vi "Engine - Generic - High Pressure Common Rail Host.vi"() -> ()   [LabVIEW 2015, in "ECS-Host.lvlib"]
uses:
  ECS-Host.lvlib
  <vilib>/addons/Software Calibration Management/XControls/SubHost.xctl
panel:
  out "RailP":sgl caption="[bar]" min=0 max=0.2 step=0.001 format="%#.3f"
  out "RailPStp":sgl caption="[bar]" min=0 max=0.2 step=0.001 format="%#.3f"
  in  "LowsideVoltageSource":enum32{"IMV PID Mode", "12V Puls Power Supply"}(ring)
  in  "_IMV/HPV Tab Control":enum32{"IMV PID", "HPV PID"}(tab)
  in  "IMV_NonPIDFF":sgl caption="[]" format="%#.2f"
  out "IMV_PIDOut":sgl caption="[]" max=50
  in  "IMV_PIDFF":sgl caption="[]" format="%#.2f"
  in  "IMV_Kp":sgl caption="[%/bar]" format="%#.2f"
  in  "IMV_Ti":sgl caption="[]" format="%#.2f"
  in  "IMV_Td":sgl caption="[]" format="%#.2f"
  in  "IMV_PIDMax":sgl caption="[%]" max=50 format="%#.2f"
  in  "IMV_PIDMin":sgl caption="[]" format="%#.2f"
  out "IMV_KpOut":sgl(slide) caption="IMV_ Kc Action" max=0 scale=0.0..100.0 scale format="%#.2f"
  out "IMV_TiOut":sgl(slide) caption="IMV_ Ti Action" max=0 scale=0.0..100.0 scale format="%#.2f"
  out "IMV_TdOut":sgl(slide) caption="IMV_ Td Action" max=0 scale=0.0..100.0 scale format="%#.2f"
  in  "HPV_NonPIDFF":sgl caption="[]" format="%#.2f"
  out "HPV_PIDOut":sgl caption="[]" max=50
  in  "HPV_PIDFF":sgl caption="[]" format="%#.2f"
  in  "HPV_Kp":sgl caption="[%/bar]" format="%#.2f"
  in  "HPV_Ti":sgl caption="[]" format="%#.2f"
  in  "HPV_Td":sgl caption="[]" format="%#.2f"
  in  "HPV_PIDMax":sgl caption="[%]" max=50 format="%#.2f"
  in  "HPV_PIDMin":sgl caption="[]" format="%#.2f"
  out "HPV_KpOut":sgl(slide) caption="HPV_ Kc_Action" max=0 scale=0.0..100.0 scale format="%#.2f"
  out "HPV_TiOut":sgl(slide) caption="IMV_ Ti Action" max=0 scale=0.0..100.0 scale format="%#.2f"
  out "HPV_TdOut":sgl(slide) caption="IMV_ Td Action" max=0 scale=0.0..100.0 scale format="%#.2f"
  in  "RPC Plot":T1(xcontrol)
  in  "IMVDutyCyc_Max":sgl caption="[]" format="%#.2f"
  in  "HPVDutyCyc_Max":sgl caption="[]" format="%#.2f"
  out "BattV":sgl caption="[]" min=0 max=0.2 step=0.001 format="%#.3f"
  out "RailP_Fault":bool
  in  "HPVDutyCyc_Man":sgl caption="[]" format="%#.2f"
  in  "IMVDutyCyc_Man":sgl caption="[]" format="%#.2f"
  in  "IMVDutyCyc_ManE":bool
  out "IMVCurrent_Calc":sgl caption="[]" min=0 max=0.2 step=0.001 format="%#.3f"
  out "IMVDutyCyc_Des":sgl=0.7671859 caption="[]" format="%#.3g"
  in  "IMVDutyCyc_Min":sgl caption="[]" format="%#.2f"
  out "IMVDutyCyc_MaxCalc":sgl caption="[]" max=50 format="%#.3g"
  in  "IMVNomResistance":sgl caption="[]" format="%#.2f"
  in  "IMVPWMFreq":sgl caption="[]" format="%#.2f"
  in  "IMVCtrl_E":bool
  in  "HPVDutyCyc_ManE":bool
  out "HPVCurrent_Calc":sgl caption="[]" min=0 max=0.2 step=0.001 format="%#.3f"
  in  "RailP_MaxThresh":sgl caption="[bar]" min=0 max=0.2 step=0.001 format="%#.3f"
  out "HPVDutyCyc_Des":sgl=0.7671859 caption="[]" format="%#.3g"
  in  "HPVDutyCyc_Min":sgl caption="[]" format="%#.2f"
  out "HPVDutyCyc_MaxCalc":sgl caption="[]" max=50 format="%#.3g"
  in  "HPVNomResistance":sgl caption="[]" format="%#.2f"
  in  "HPVPWMFreq":sgl caption="[Hz]" format="%#.2f"
  in  "HPVCtrl_E":bool
  in  "RailPControlMode":enum32{"IMV PID Mode", "HPV PID Mode"}(ring)
  in  "HPCR_FaultClear":bool
  # "+"
  # "+"
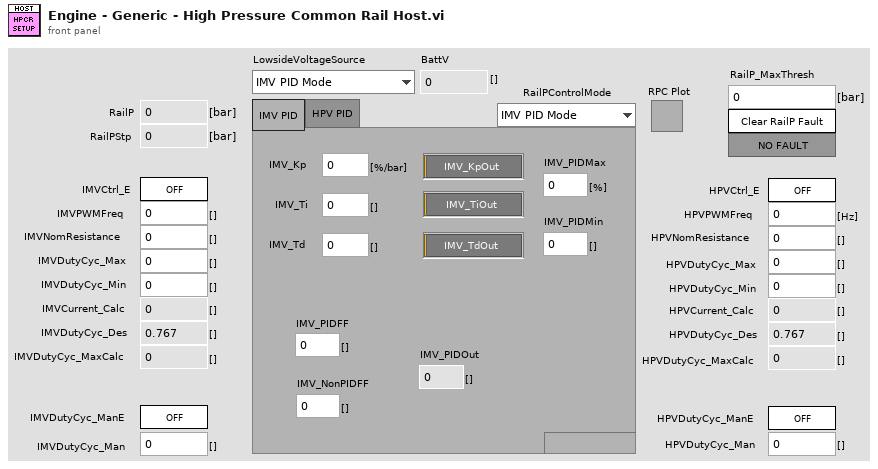
[diagram p1: front panel]
types:
  T1 = cluster{"Name":string, "Host VI":path, "Pairing File":path, "Display Name":string}
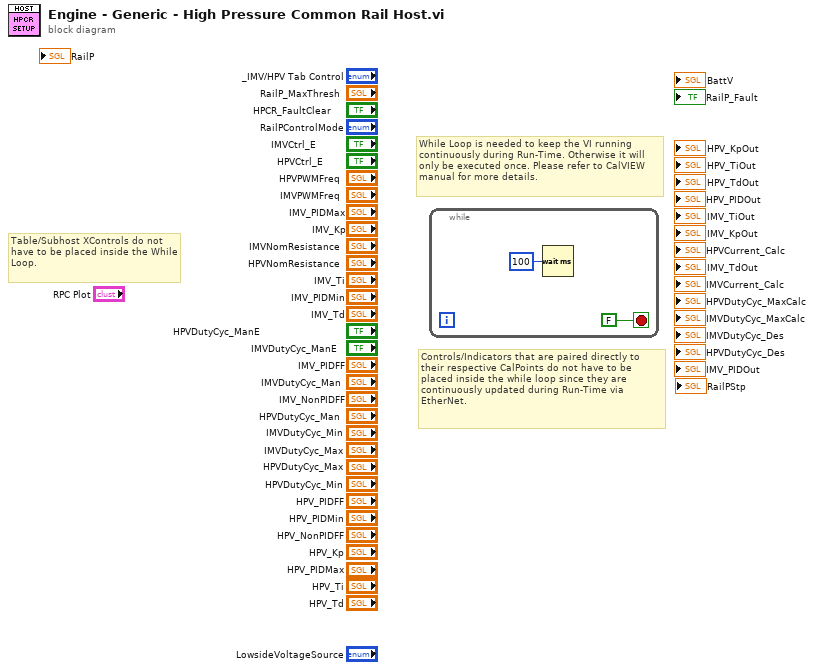
[diagram p0: block diagram]
diagram:
  # "Table/Subhost XControls do not have to be placed inside the While Loop."
  # "While Loop is needed to keep the VI running\ncontinuously during Run-Time. Otherwise it will only be executed once. Please refer to CalVIEW manual for more details."
  # "Controls/Indicators that are paired directly to their respective CalPoints do not have to be placed inside the while loop since they are continuously updated during Run-Time via EtherNet."
  n1 = while {
    stop <- FALSE stop-if-true
    n2 = Wait (ms)(milliseconds to wait=u32 100) -> ()  [unwired: 1 out]
  }
